vi "RP recorder.vi"(8 "Error In":errorcluster, 10 "Server port":u16=1002, 11 "Server address":string="192.168.1.100") -> (0 "Error Out":errorcluster)   [LabVIEW 2015]
uses:
  Mode.ctl
  RP Command.ctl
  File/Controls/File formats.ctl
panel:
  out "Server  output":string
  in  "Start server":bool
  out "Record start pos":u32=1
  in  "Trigger offset":i32=-100000 format="0x%x (%d)"
  in  "Read subset":bool
  out "Data File  Path":path
  in  "Auto-save file":bool=TRUE
  out "Trigger state":bool
  in  "Read trigger":bool=TRUE
  in  "FPGA Logic":enum16{"Digitizer", "Fast Digitizer"}(ring)
  in  "Post-trigger samples":u64=11534336 format="0x%x (%d)"
  in  "Trigger":bool
  in  "Read":bool
  in  "Arm":bool
  in  "Desimation rate":u64=125
  out "Temperature Chart":dbl(graph)=48.847186279148
  out "Thermometer":dbl(slide)=48.847186279148 scale=0.0..100.0
  in  "Read Temperature":bool=TRUE
  in  "Status offset":u64=8 format="%x"
  in  "Ranges":dbl[](array[numeric])=[20.0, 1.0]
  out "x-y":u32=4294967295
  out "element":u32
  out "Phase  Graph":u32[](graph)
  in  "Mode":T1=enum."Digitizer"
  out "Status response":u32=1
  in  "Status":bool
  out "Waveform Graph":sgl[][](graph)
  in  "Record":bool
  in  "Stop Server":bool
  out "bytes written":i32=8
  in  "Process Stop Button":bool
  out "Phase increment":u64=1717987
  in  "Output frequency":dbl=50000.0 format="%#_6p"
  in  "Samples to read":u64=67108864 format="0x%x (%d)"
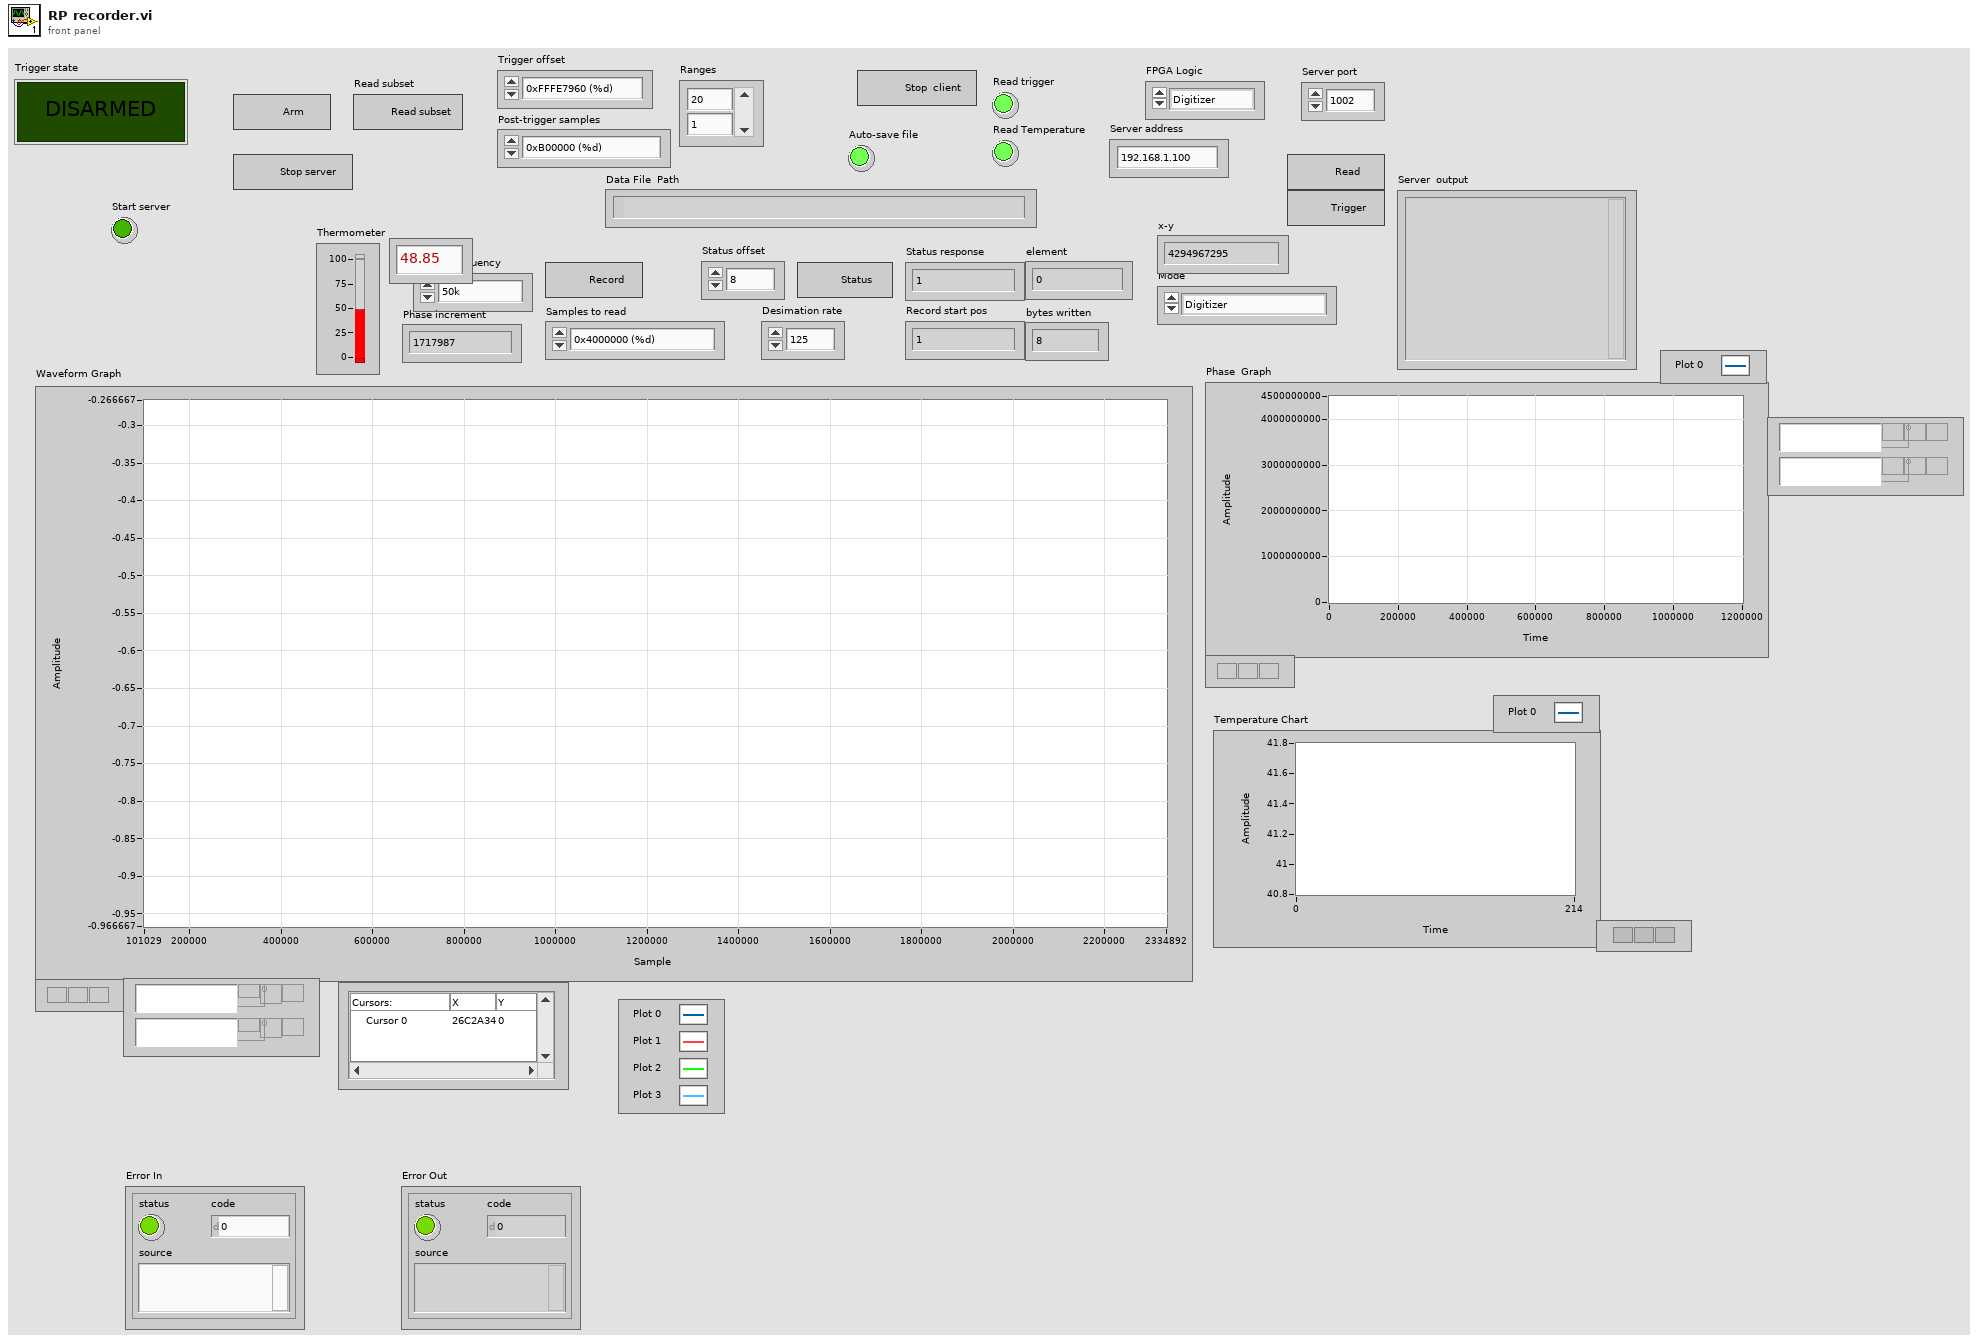
[diagram p1: front panel]
types:
  T1 = typedef "Mode.ctl" = enum16{"Filter", "Lockin test", "Snapshot test", "Digitizer"}
  T2 = enum16{"big-endian, network order", "native, host order", "little-endian"}
  T3 = typedef "RP Command.ctl" = enum16{"Set frequency", "Arm and get data", "Stop server", "Get status", "Get temperature", "Set decimation", "Arm", "Software trigger", "Get whole buffer", "Get chunk", "System call", "Get config", "Set config", "Read FIFO", "Play pattern", "Set frequency batch"}
  T4 = typedef "File formats.ctl" = enum16{"TDMS", "ASCII", "BINARY"}
  T5 = typedef "RP info.ctl" = cluster{"Range":dbl, "Name":string, "waveform period":dbl, "waveform start":dbl, "Frequency":u32, "Phase":u32}
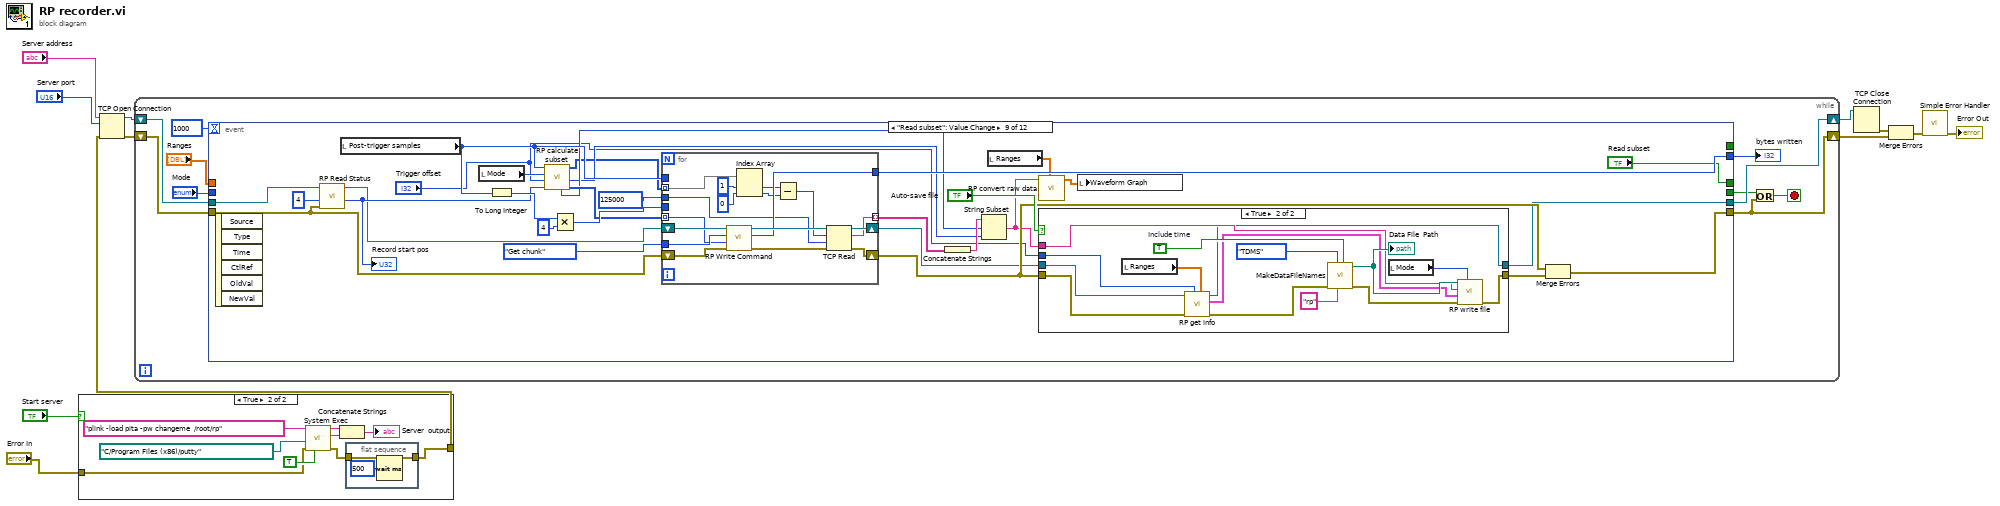
[diagram p0: block diagram]
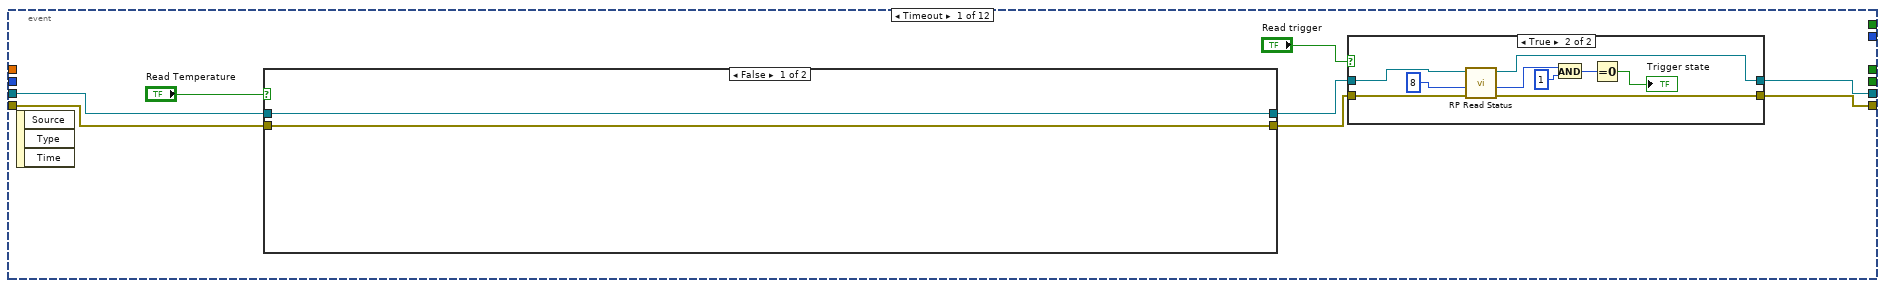
[diagram p3: hidden frame]
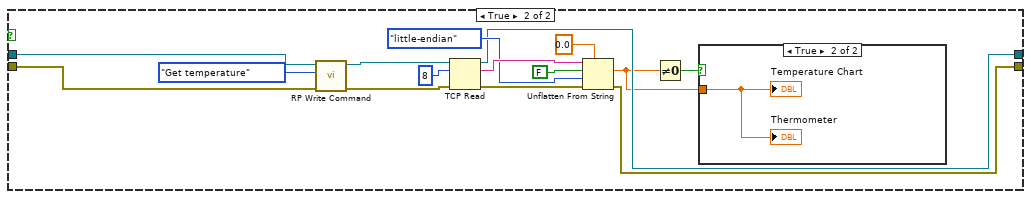
[diagram p5: hidden frame]
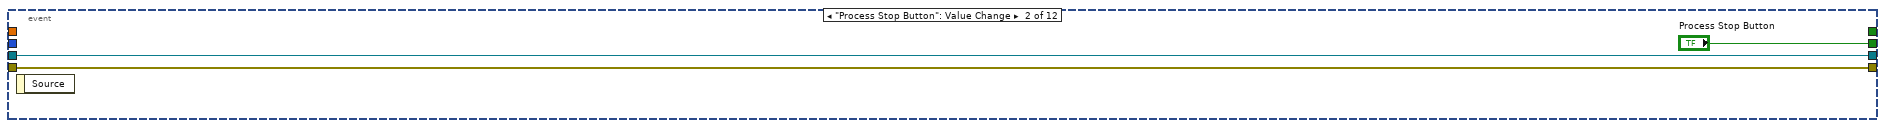
[diagram p7: hidden frame]
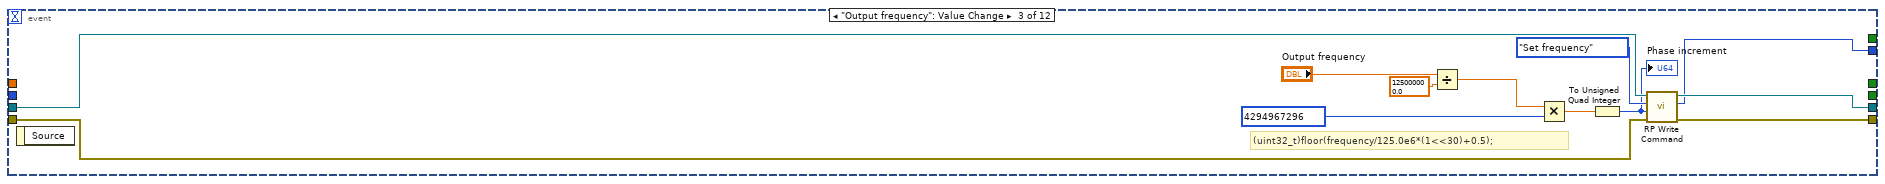
[diagram p8: hidden frame]
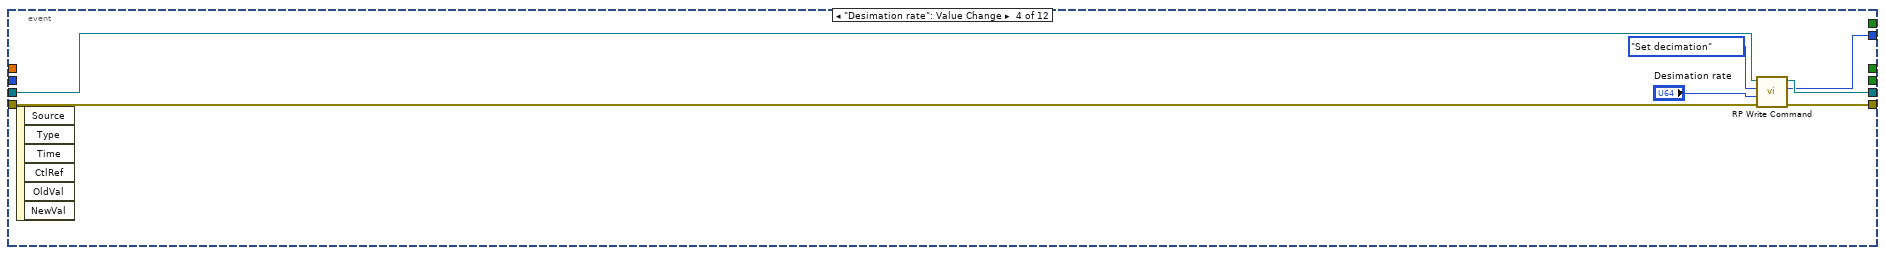
[diagram p9: hidden frame]
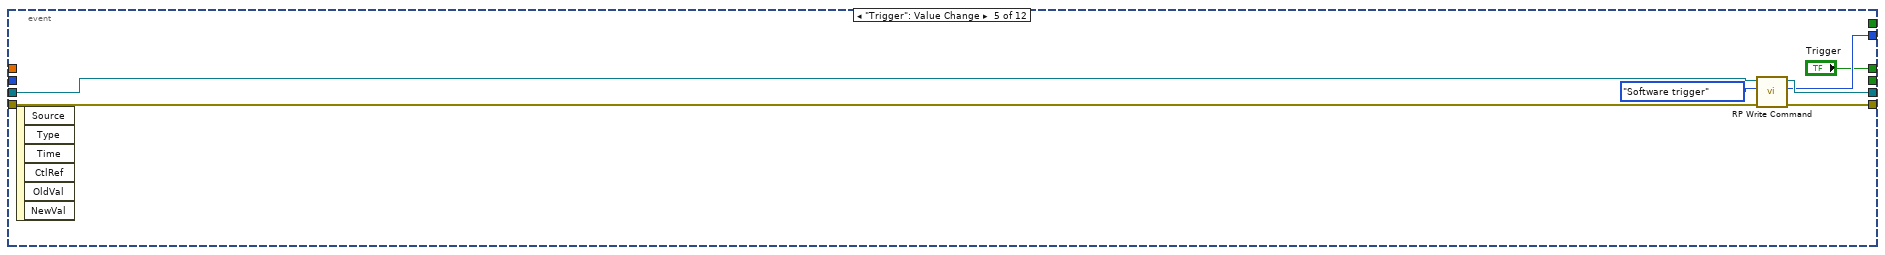
[diagram p10: hidden frame]
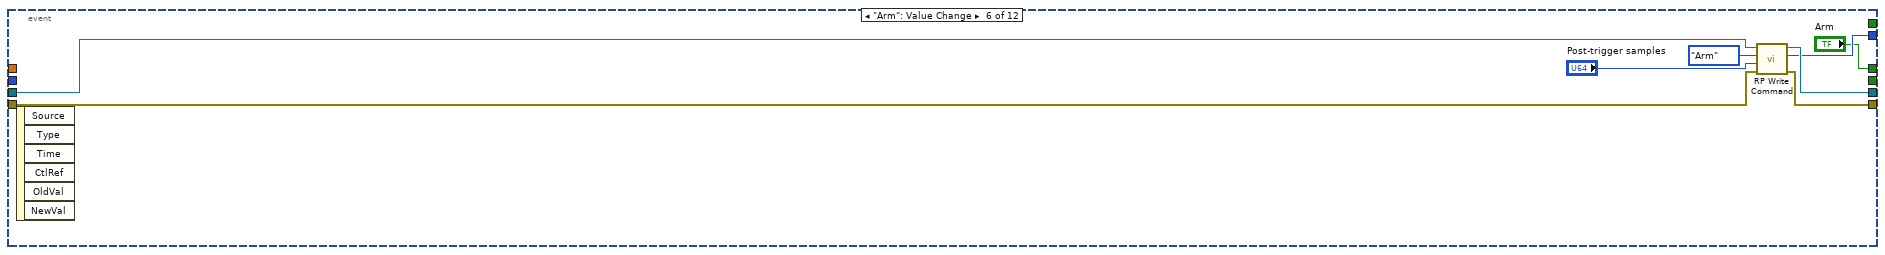
[diagram p11: hidden frame]
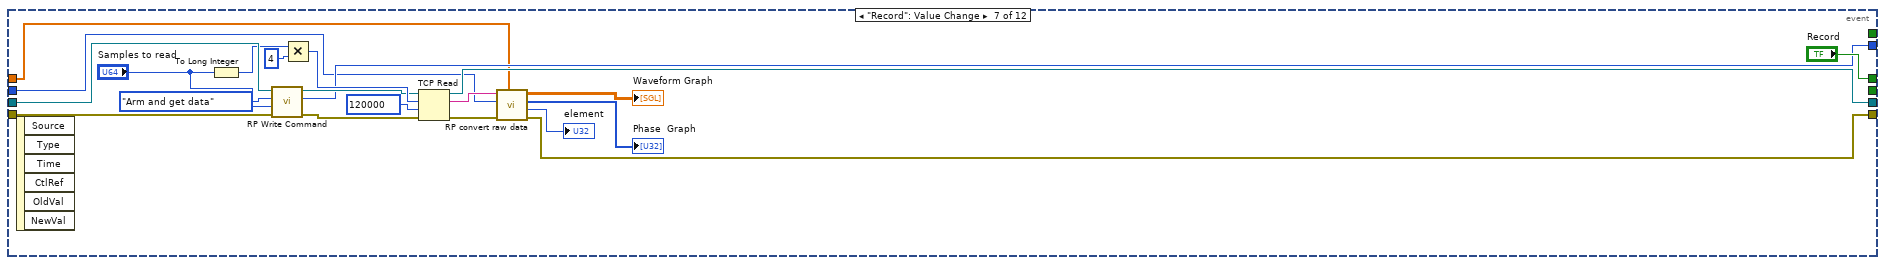
[diagram p12: hidden frame]
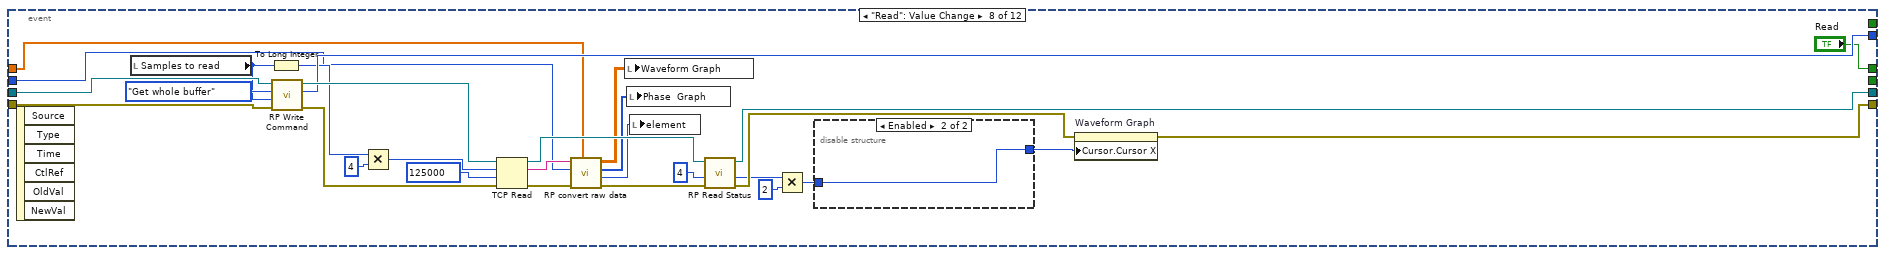
[diagram p13: hidden frame]
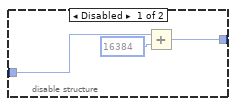
[diagram p14: hidden frame]
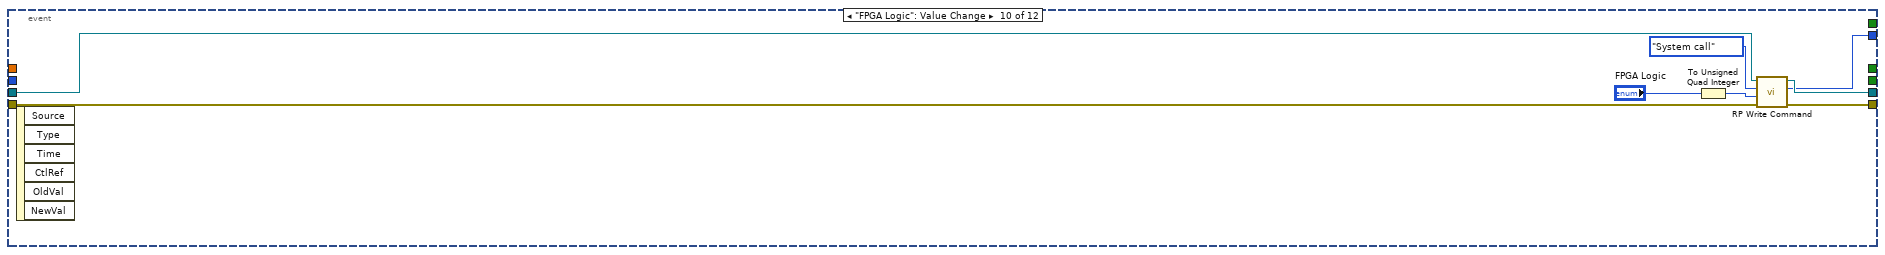
[diagram p16: hidden frame]
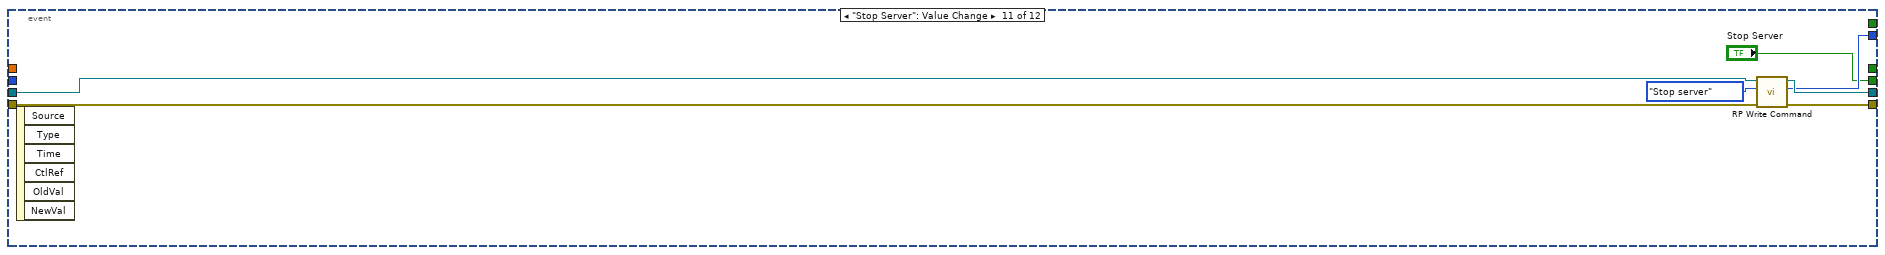
[diagram p17: hidden frame]
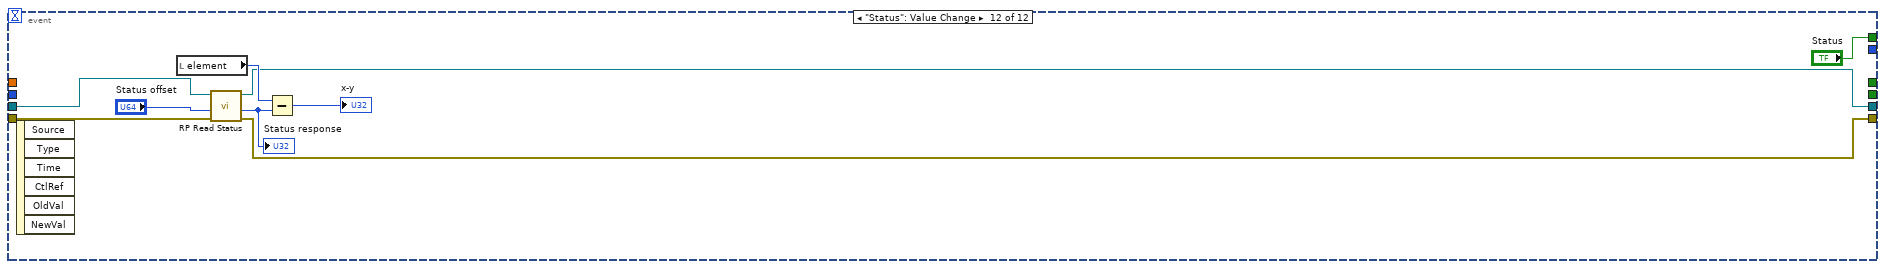
[diagram p18: hidden frame]
diagram:
  n1 = case shown="True" "Start server" {
    tunnel: [w13 w14] -> w2
    tunnel: "Error In" -> [w13 w16]
    frame False {
    }
    frame True {
      n2 = call <vilib>:"System Exec.vi"("run minimized? (F)"=TRUE, "error in (no error)"=w16, "working directory"=path "C:/Program Files (x86)/putty", "command line"="plink -load pita -pw changeme  /root/rp") -> ("error out"=w15:errorcluster, "standard error"=w18:string, "standard output"=w22:string)  [unwired: 4 in, 1 out]
      n3 = Concatenate Strings(w22, w18) -> (→"Server  output":string)
      n4 = flat-sequence {
        tunnel: w15 -> [w24]
        tunnel: [w24] -> w14
        frame #0 {
          n5 = Wait (ms)(milliseconds to wait=u32 500) -> ()  [unwired: 1 out]
        }
      }
    }
  }
  n6 = TCP Open Connection(address="Server address", remote port or service name="Server port", error in (no error)=w2) -> (connection ID=w7:refnum<k5>, error out=w8:errorcluster)  [unwired: 2 in]
  n7 = while {
    shift-right: [w32] -> w6
    shift-left: w7 -> [w33]
    shift-right: [w30] -> w5
    shift-left: w8 -> [w34]
    stop <- w28 stop-if-true
    n8 = event shown="[8] \"Read subset\": Value Change" {
      selector: _ -> [_ _ _ _ _ _ _ _ _ _ _ _]
      dyn-events: _ -> [_ _ _ _ _ _ _ _ _ _ _ _]
      timeout: 1000 -> [_ _ _ _ _ _ _ _ _ _ _ _]
      tunnel: w34 -> [w40 w73 w81 w93 w100 w108 w122 w153 w176 w234 w241 w247]
      tunnel: w33 -> [w41 w72 w80 w92 w99 w107 w125 w156 w178 w233 w239 w243]
      tunnel: [w36 w73 w76 w89 w96 w104 w113 w150 w183 w229 w238 w246] -> w30
      tunnel: [w35 w72 w77 w90 w97 w105 w127 w146 w166 w228 w237 w244] -> w32
      tunnel: [_ "Process Stop Button" _ _ _ _ _ _ _ _ "Stop Server" _] -> w29
      tunnel: [_ _ _ _ _ _ _ _ _ _ _ "Status"] -> _
      tunnel: [_ _ w75 w88 w95 w103 w120 w151 w189 w227 w236 _] -> w31
      tunnel: [_ _ _ _ "Trigger" "Arm" "Record" "Read" "Read subset" _ _ _] -> _
      tunnel: "Ranges" -> [_ _ _ _ _ _ w109 w143 _ _ _ _]
      tunnel: "Mode" -> [_ _ _ _ _ _ w110 w130 _ _ _ _]
      event Timeout {
        n9 = event-data() -> ()  [unwired: 1 in, 3 out]
        n10 = case shown="False" "Read Temperature" {
          tunnel: w41 -> [w55 w70]
          tunnel: w40 -> [w54 w69]
          tunnel: [w55 w58] -> w38
          tunnel: [w54 w60] -> w37
          frame False {
          }
          frame True {
            n11 = call "RP Write Command.vi"("Error In"=w69, "Command number"=RP_Command."Get temperature", "connection ID"=w70) -> ("Error Out"=w61:errorcluster, "connection ID out"=w59:refnum<k5>)  [unwired: 6 in, 1 out]
            n12 = TCP Read(connection ID=w59, bytes to read=8, error in (no error)=w61) -> (connection ID out=w58:refnum<k5>, data out=w67:string, error out=w65:errorcluster)  [unwired: 2 in]
            n13 = Unflatten From String(type=0.0, binary string=w67, data includes array or string size? (T)=FALSE, byte order (0:big-endian, network order)=T2."little-endian", error in (no error)=w65) -> (value=w57:dbl, error out=w60:errorcluster)  [unwired: 1 out]
            n14 = Not Equal To 0?(x=w57) -> (x != 0?=w56:bool)
            n15 = case shown="True" w56 {
              tunnel: w57 -> [_ w71]
              frame False {
              }
              frame True {
                "Thermometer" <- w71
                "Temperature Chart" <- w71
              }
            }
          }
        }
        n16 = case shown="True" "Read trigger" {
          tunnel: w38 -> [w43 w52]
          tunnel: w37 -> [w44 w53]
          tunnel: [w44 w48] -> w36
          tunnel: [w43 w45] -> w35
          frame False {
          }
          frame True {
            n17 = call "RP Read Status.vi"("Error In"=w53, "Status offset"=u64 8, "connection ID"=w52) -> ("Error Out"=w48:errorcluster, "Status response"=w50:u32, "connection ID out"=w45:refnum<k5>)  [unwired: 6 in]
            n18 = And(x=w50, y=u32 1) -> (x .and. y?=w47:u32)
            n19 = Equal To 0?(x=w47) -> (x = 0?=→"Trigger state":bool)
          }
        }
      }
      event "Process Stop Button": Value Change {
        n20 = event-data() -> ()  [unwired: 1 in, 1 out]
      }
      event "Output frequency": Value Change {
        # "(uint32_t)floor(frequency/125.0e6*(1<<30)+0.5);"
        n21 = event-data() -> ()  [unwired: 1 in, 1 out]
        n22 = Divide(x="Output frequency", y=125000000.0) -> (x/y=w83:dbl)
        n23 = Multiply(x=w83, y=i64 4294967296) -> (x*y=w82:dbl)
        n24 = To Unsigned Quad Integer(1:w82) -> (0:w78:u64)
        "Phase increment" <- w78
        n25 = call "RP Write Command.vi"("Error In"=w81, "Command payload"=w78, "Command number"=RP_Command."Set frequency", "connection ID"=w80) -> ("Error Out"=w76:errorcluster, "bytes written"=w75:i32, "connection ID out"=w77:refnum<k5>)  [unwired: 5 in]
      }
      event "Desimation rate": Value Change {
        n26 = event-data() -> ()  [unwired: 1 in, 6 out]
        n27 = call "RP Write Command.vi"("Error In"=w93, "Command payload"="Desimation rate", "Command number"=RP_Command."Set decimation", "connection ID"=w92) -> ("Error Out"=w89:errorcluster, "bytes written"=w88:i32, "connection ID out"=w90:refnum<k5>)  [unwired: 5 in]
      }
      event "Trigger": Value Change {
        n28 = event-data() -> ()  [unwired: 1 in, 6 out]
        n29 = call "RP Write Command.vi"("Error In"=w100, "Command number"=RP_Command."Software trigger", "connection ID"=w99) -> ("Error Out"=w96:errorcluster, "bytes written"=w95:i32, "connection ID out"=w97:refnum<k5>)  [unwired: 6 in]
      }
      event "Arm": Value Change {
        n30 = event-data() -> ()  [unwired: 1 in, 6 out]
        n31 = call "RP Write Command.vi"("Error In"=w108, "Command payload"="Post-trigger samples", "Command number"=RP_Command."Arm", "connection ID"=w107) -> ("Error Out"=w104:errorcluster, "bytes written"=w103:i32, "connection ID out"=w105:refnum<k5>)  [unwired: 5 in]
      }
      event "Record": Value Change {
        n32 = event-data() -> ()  [unwired: 1 in, 6 out]
        n33 = To Long Integer(number="Samples to read") -> (32bit integer=w119:i32)
        n34 = call "RP Write Command.vi"("Error In"=w122, "Command payload"="Samples to read", "Command number"=RP_Command."Arm and get data", "connection ID"=w125) -> ("Error Out"=w121:errorcluster, "bytes written"=w120:i32, "connection ID out"=w123:refnum<k5>)  [unwired: 5 in]
        n35 = Multiply(x=w119, y=4) -> (x*y=w126:i32)
        n36 = TCP Read(connection ID=w123, bytes to read=w126, error in (no error)=w121, 9:120000 ("timeout ms (25000)")) -> (connection ID out=w127:refnum<k5>, data out=w116:string, error out=w114:errorcluster)  [unwired: 1 in]
        n37 = call "RP convert raw data.vi"("Max Volts"=w109, "Error In"=w114, "Format"=w110, "data stream"=w116) -> ("Error Out"=w113:errorcluster, "element"=→"element":u32, "phase out"=→"Phase  Graph":u32[], "data out"=→"Waveform Graph":sgl[][])  [unwired: 4 in]
      }
      event "Read": Value Change {
        n38 = event-data() -> ()  [unwired: 1 in, 6 out]
        n39 = local read "Samples to read"() -> (w145:u64)
        n40 = To Long Integer(number=w145) -> (32bit integer=w148:i32)
        n41 = call "RP Write Command.vi"("Error In"=w153, "Command payload"=w145, "Command number"=RP_Command."Get whole buffer", "connection ID"=w156) -> ("Error Out"=w152:errorcluster, "bytes written"=w151:i32, "connection ID out"=w154:refnum<k5>)  [unwired: 5 in]
        n42 = Multiply(x=w148, y=4) -> (x*y=w157:i32)
        n43 = TCP Read(connection ID=w154, bytes to read=w157, error in (no error)=w152, 9:125000 ("timeout ms (25000)")) -> (connection ID out=w147:refnum<k5>, data out=w142:string, error out=w132:errorcluster)  [unwired: 1 in]
        n44 = call "RP convert raw data.vi"("Max Volts"=w143, "Error In"=w132, "Format"=w130, "data stream"=w142) -> ("Error Out"=w131:errorcluster, "element"=w139:u32, "phase out"=w140:u32[], "data out"=w141:sgl[][])  [unwired: 4 in]
        n45 = local write "Waveform Graph"(w141) -> ()
        n46 = local write "Phase  Graph"(w140) -> ()
        n47 = local write "element"(w139) -> ()
        n48 = call "RP Read Status.vi"("Error In"=w131, "Status offset"=u64 4, "connection ID"=w147) -> ("Error Out"=w137:errorcluster, "Status response"=w136:u32, "connection ID out"=w146:refnum<k5>)  [unwired: 6 in]
        n49 = Multiply(x=w136, y=u32 2) -> (x*y=w134:u32)
        n50 = disable-structure shown="Enabled" {
          disable-tunnel: w134 -> [w161 w162]
          disable-tunnel: [w159 w162] -> w133
          frame Disabled {
            n51 = Add(x=w161, y=16384) -> (x+y=w159:u32)
          }
          frame Enabled {
          }
        }
        n52 = property on="Waveform Graph" class="WFGraph (strict)"(error in=w137, "Cursor.Cursor X"=w133) -> (error out=w150:errorcluster)  [unwired: 1 in, 1 out]
      }
      event "Read subset": Value Change {
        n53 = event-data() -> ()  [unwired: 1 in, 6 out]
        n54 = call "RP Read Status.vi"("Error In"=w176, "Status offset"=u64 4, "connection ID"=w178) -> ("Status response"=w175:u32, "connection ID out"=w174:refnum<k5>)  [unwired: 6 in, 1 out]
        "Record start pos" <- w175
        n55 = local read "Post-trigger samples"() -> (w180:u64)
        n56 = local read "Mode"() -> (w179:T1)
        n57 = To Long Integer(number=w180) -> (32bit integer=w188:i32)
        n58 = call "RP calculate subset.vi"("Record start position"=w175, "Trigger offset"="Trigger offset", "Mode"=w179, "Post-trigger samples"=w180) -> ("Merged subsets"=w173:u64[], "record length"=w169:i32, "Subsets"=w163:i32[][], "pre-trigger trim"=w170:i32)  [unwired: 4 in]
        n59 = Multiply(x=w188, y=4) -> (x*y=w191:i32)
        n60 = for {
          tunnel: w191 -> [_]
          tunnel: RP_Command."Get chunk" ("Command number") -> [w209]
          tunnel: [w206] -> w189
          tunnel: 125000 ("timeout ms (25000)") -> [w204]
          tunnel: w180 -> [_]
          shift-right: [w203] -> w184
          shift-left: w176 -> [w202]
          shift-right: [w205] -> w167
          shift-left: w174 -> [w201]
          tunnel: w173 -> [w200] mode=indexing
          tunnel: [w199] -> w172 mode=indexing
          tunnel: w163 -> [w197] mode=indexing
          n61 = call "RP Write Command.vi"("Error In"=w202, "Command payload"=w200, "Command number"=w209, "connection ID"=w201) -> ("Error Out"=w207:errorcluster, "bytes written"=w206:i32, "connection ID out"=w208:refnum<k5>)  [unwired: 5 in]
          n62 = Index Array(array=w197, index #1=1 ("index"), index #2=0 ("index")) -> (element #1=w196:i32, element #2=w195:i32)
          n63 = Subtract(x=w196, y=w195) -> (x-y=w194:i32)
          n64 = TCP Read(connection ID=w208, bytes to read=w194, error in (no error)=w207, 9:w204) -> (connection ID out=w205:refnum<k5>, data out=w199:string, error out=w203:errorcluster)  [unwired: 1 in]
        }
        n65 = Concatenate Strings(w172) -> (w171:string)
        n66 = String Subset(string=w171, offset (0)=w170, length (rest)=w169) -> (substring=w168:string)
        n67 = local read "Ranges"() -> (w164:dbl[])
        n68 = call "RP convert raw data.vi"("Max Volts"=w164, "data stream"=w168) -> ("data out"=w181:sgl[][])  [unwired: 6 in, 3 out]
        n69 = case shown="True" "Auto-save file" {
          tunnel: w184 -> [w211 w219]
          tunnel: w168 -> [_ w222]
          tunnel: [w211 w220] -> w182
          tunnel: w167 -> [w210 w217]
          tunnel: [w210 w216] -> w166
          tunnel: "Trigger offset" -> [_ w214]
          frame False {
          }
          frame True {
            w224 = TRUE  # Include time
            n70 = local read "Ranges"() -> (w215:dbl[])
            n71 = call "RP get info.vi"("Ranges"=w215, "Trigger offset"=w214, "Error In"=w219, "connection ID"=w217) -> ("Error Out"=w218:errorcluster, "Channel info"=w213:T5[], "connection ID out"=w216:refnum<k5>)  [unwired: 5 in]
            n72 = call "MakeDataFileNames.vi"("Include time"=w224, "File Prefix"="rp", "File format"=File_formats."TDMS", "Error In"=w218) -> ("Error Out"=w221:errorcluster, "Data File  Path"=w223:path)  [unwired: 4 in, 2 out]
            "Data File  Path" <- w223
            n73 = local read "Mode"() -> (w212:T1)
            n74 = call "RP write file.vi"("Mode"=w212, "Error In"=w221, "Channel info"=w213, "Data"=w222, "File Path"=w223) -> ("Error Out"=w220:errorcluster)  [unwired: 4 in, 2 out]
          }
        }
        n75 = local write "Waveform Graph"(w181) -> ()
        n76 = Merge Errors(w184, w182) -> (w183:errorcluster)
      }
      event "FPGA Logic": Value Change {
        n77 = event-data() -> ()  [unwired: 1 in, 6 out]
        n78 = To Unsigned Quad Integer(1:"FPGA Logic") -> (0:w231:u64)
        n79 = call "RP Write Command.vi"("Error In"=w234, "Command payload"=w231, "Command number"=RP_Command."System call", "connection ID"=w233) -> ("Error Out"=w229:errorcluster, "bytes written"=w227:i32, "connection ID out"=w228:refnum<k5>)  [unwired: 5 in]
      }
      event "Stop Server": Value Change {
        n80 = event-data() -> ()  [unwired: 1 in, 6 out]
        n81 = call "RP Write Command.vi"("Error In"=w241, "Command number"=RP_Command."Stop server", "connection ID"=w239) -> ("Error Out"=w238:errorcluster, "bytes written"=w236:i32, "connection ID out"=w237:refnum<k5>)  [unwired: 6 in]
      }
      event "Status": Value Change {
        n82 = event-data() -> ()  [unwired: 1 in, 6 out]
        n83 = local read "element"() -> (w249:u32)
        n84 = call "RP Read Status.vi"("Error In"=w247, "Status offset"="Status offset", "connection ID"=w243) -> ("Error Out"=w246:errorcluster, "Status response"=w245:u32, "connection ID out"=w244:refnum<k5>)  [unwired: 6 in]
        "Status response" <- w245
        n85 = Subtract(x=w249, y=w245) -> (x-y=→"x-y":u32)
      }
    }
    "bytes written" <- w31
    n86 = Or(x=w29, y=w30) -> (x .or. y?=w28:bool)
  }
  n87 = TCP Close Connection(connection ID=w6) -> (error out=w10:errorcluster)  [unwired: 2 in, 1 out]
  n88 = Merge Errors(w10, w5) -> (w9:errorcluster)
  n89 = call <vilib>:"Simple Error Handler.vi"("error in (no error)"=w9) -> ("error out"=→"Error Out":errorcluster)  [unwired: 4 in, 4 out]
